vi "Elevator Read Encoder.vi"(11 "Reset Encoders":bool) -> (3 "Encoder Values":T1)   [LabVIEW 2017]
uses:
  Common Code/Encoder Values.ctl
  Public/Documents/Cross The Road Electronics/Phoenix-LabVIEW/Motor Controller/Get/CTRE_Phoenix_MotorController_GetSelectedSensorData.vi
  Public/Documents/Cross The Road Electronics/Phoenix-LabVIEW/Motor Controller/Get/CTRE_Phoenix_MotorController_GetOutputCurrent_Enhanced.vi
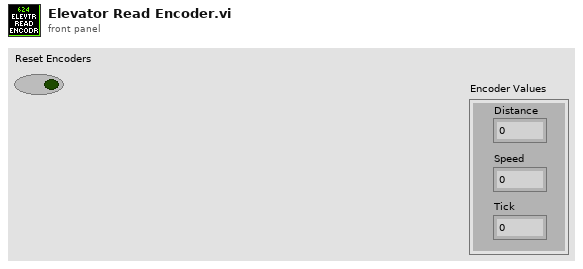
[diagram p1: front panel]
types:
  T1 = typedef "Encoder Values.ctl" = cluster{"Distance":dbl, "Speed":dbl, "Tick":dbl}
  T2 = typedef "WPI_MotorControlDeviceRef.ctl" = cluster{"DeviceStatus":errorcluster, "Type":T3, "PWM":cluster{"PWM Channel":T4, "DeadBand":T5}, "CAN":cluster{"Device Number":u8, "SetOutput VI Ref":variant, "GetOutput VI Ref":variant, "Enable VI Ref":variant, "Disable VI Ref":variant, "Data":variant}, "Invert":bool, "DIO PWM":cluster{"PWM \"Enable\" Channel":T4, "DIOChannel":T6, "PWM Rate":dbl}}
  T3 = typedef "WPI_MotorControlType.ctl" = enum16{"PWM", "CAN", "DIO PWM"}
  T4 = typedef "FPGA_DIOPWMChannel.ctl" = enum8{"PWM 0", "PWM 1", "PWM 2", "PWM 3", "PWM 4", "PWM 5", "PWM 6", "PWM 7", "PWM 8", "PWM 9", "PWM MXP 0", "PWM MXP 1", "PWM MXP 2", "PWM MXP 3", "PWM MXP 4", "PWM MXP 5", "PWM MXP 6", "PWM MXP 7", "PWM MXP 8", "PWM MXP 9", "Invalid"}
  T5 = typedef "WPI_PWMDeadband.ctl" = cluster{"Name":string, "maxPositivePwm":i32, "minPositivePwm":i32, "centerPwm":i32, "maxNegativePwm":i32, "minNegativePwm":i32, "angularRange":u16}
  T6 = typedef "FPGA_DIOChannel.ctl" = enum8{"DIO 0", "DIO 1", "DIO 2", "DIO 3", "DIO 4", "DIO 5", "DIO 6", "DIO 7", "DIO 8", "DIO 9", "DIO MXP 0", "DIO MXP 1", "DIO MXP 2", "DIO MXP 3", "DIO MXP 4", "DIO MXP 5", "DIO MXP 6", "DIO MXP 7", "DIO MXP 8", "DIO MXP 9", "DIO MXP 10", "DIO MXP 11", "DIO MXP 12", "DIO MXP 13", "DIO MXP 14", "DIO MXP 15", "SPI Port CS1", "SPI Port CS2", "SPI Port CS3", "SPI Port MISO", "SPI Port MOSI", "Invalid"}
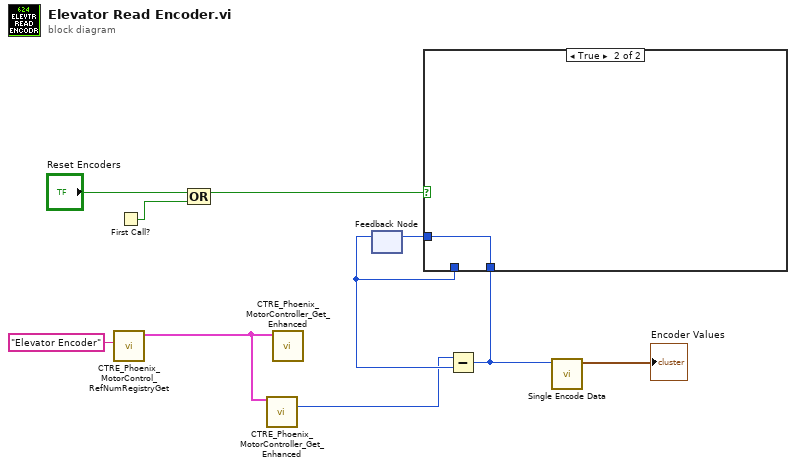
[diagram p0: block diagram]
diagram:
  n1 = call "CTRE_Phoenix_MotorControl_RefNumRegistryGet.vi"("refnum name"="Elevator Encoder") -> ("PhoenixMotorControlDevRef"=w8:T2)  [unwired: 9 in, 1 out]
  n2 = First Call?() -> (First Call?: T/F=w4:bool)
  n3 = Compound Arithmetic op=OR("Reset Encoders", w4) -> (w5:bool)
  n4 = call-poly "CTRE_Phoenix_MotorController_Get_Enhanced.vi"("PhoenixMotorControlDevRef"=w8) -> ("Position (Raw Sensor Units)"=w1:i32)  [unwired: 11 in, 3 out]
  n5 = call-poly "CTRE_Phoenix_MotorController_Get_Enhanced.vi"("PhoenixMotorControlDevRef"=w8) -> ()  [unwired: 12 in, 3 out]
  n6 = feedback #1() -> (w2:i32)  [unwired: 1 in]
  n7 = Subtract(x=w1, y=w2) -> (x-y=w3:i32)
  n8 = case shown="True" w5 {
    tunnel: [w11 w12] -> w7
    tunnel: w2 -> [w11 _]
    tunnel: w3 -> [_ w12]
    frame False {
    }
    frame True {
    }
  }
  n9 = feedback-in #1(w7) -> ()
  n10 = call "Single Encode Data.vi"("Distance"=w3) -> ("Encoder Values"=→"Encoder Values":T1)  [unwired: 10 in]
